vi "Is VI Server Required.vi"(8 "error in (no error)":errorcluster, 11 "Boolean Assertion in":refnum<class "Boolean Assertion.lvclass">) -> (0 "error out":errorcluster, 2 "VI Server Required?":bool, 3 "Boolean Assertion out":refnum<class "Boolean Assertion.lvclass">)   [LabVIEW 2020, in "MacroAssert.lvlib" / "Boolean Assertion.lvclass"]
doc: "Outputs whether VI Server is required to perform the given step."
uses:
  Boolean Assertion.lvclass
  Boolean Assertion.lvclass/Boolean Assertion.ctl
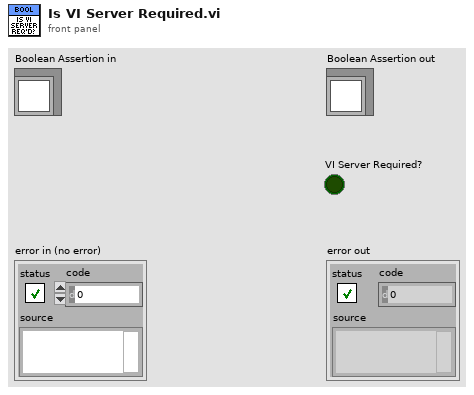
[diagram p1: front panel]
types:
  T1 = typedef "MacroAssert.lvlib/Boolean Assertion.lvclass/Boolean Assertion Type.ctl" = enum16{"Boolean Ctl Value", "Ctl Visible Property", "Ctl is Enabled", "Ctl is Grayed Out", "Ctl Key Focus Property", "VI Front Panel is Open", "Window is in Running Windows", "Window is in Monitor Bounds"}
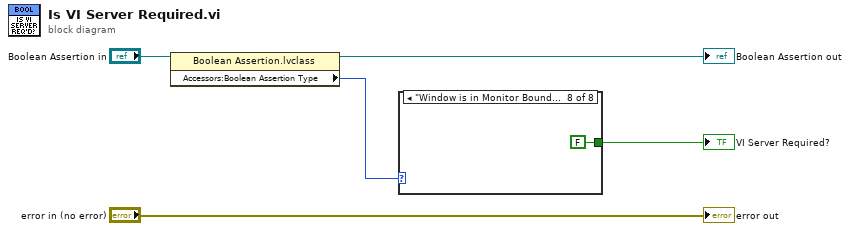
[diagram p0: block diagram]
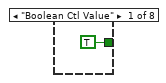
[diagram p2: hidden frame]
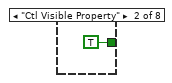
[diagram p3: hidden frame]
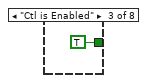
[diagram p4: hidden frame]
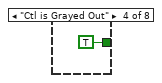
[diagram p5: hidden frame]
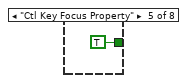
[diagram p6: hidden frame]
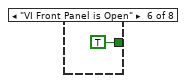
[diagram p7: hidden frame]
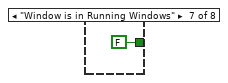
[diagram p8: hidden frame]
diagram:
  n1 = property class="Boolean Assertion.lvclass"(reference="Boolean Assertion in") -> (reference out=→"Boolean Assertion out":refnum<class "Boolean Assertion.lvclass">, "Accessors:Boolean Assertion Type"=w3:T1)  [unwired: 1 in, 1 out]
  n2 = case shown="\"Window is in Monitor Bounds\"" w3 {
    tunnel: [TRUE TRUE TRUE TRUE TRUE TRUE FALSE FALSE] -> w2
    frame "Boolean Ctl Value" {
    }
    frame "Ctl Visible Property" {
    }
    frame "Ctl is Enabled" {
    }
    frame "Ctl is Grayed Out" {
    }
    frame "Ctl Key Focus Property" {
    }
    frame "VI Front Panel is Open" {
    }
    frame "Window is in Running Windows" {
    }
    frame "Window is in Monitor Bounds" {
    }
  }
  "VI Server Required?" <- w2
  "error out" <- "error in (no error)"
